vi "Test Script.vi"() -> ()   [LabVIEW 2016, in "PostBuildSupport.lvclass"]
uses:
  PostBuildSupport.lvclass
  PostBuildSupport.lvclass/PostBuildSupport.ctl
panel:
  in  "Output Package File Path":path
  in  "Product Name":string="Multichannel Lockin"
  in  "Package Version":string="2.8.9.18"
  in  "Package Source Folder":path=path "C:/user/patrick/git/Multichannel-Lockin/src"
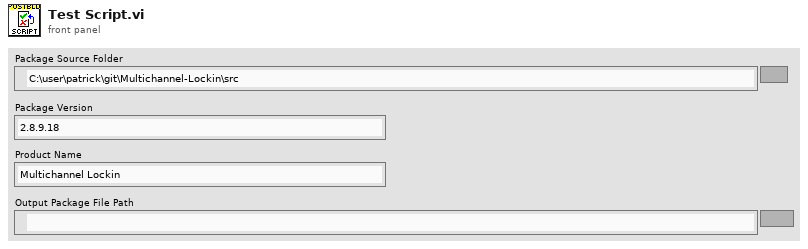
[diagram p1: front panel]
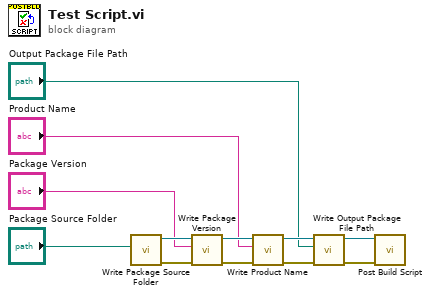
[diagram p0: block diagram]
diagram:
  n1 = call "Write Package Source Folder.vi"("Package Source Folder"="Package Source Folder") -> ("error out"=w11:errorcluster, "PostBuildSupport out"=w12:refnum<class "PostBuildSupport.lvclass">)  [unwired: 9 in]
  n2 = call "Write Package Version.vi"("error in (no error)"=w11, "Package Version"="Package Version", "PostBuildSupport in"=w12) -> ("error out"=w9:errorcluster, "PostBuildSupport out"=w10:refnum<class "PostBuildSupport.lvclass">)  [unwired: 7 in]
  n3 = call "Write Product Name.vi"("error in (no error)"=w9, "Product Name"="Product Name", "PostBuildSupport in"=w10) -> ("error out"=w7:errorcluster, "PostBuildSupport out"=w8:refnum<class "PostBuildSupport.lvclass">)  [unwired: 7 in]
  n4 = call "Write Output Package File Path.vi"("error in (no error)"=w7, "Output Package File Path"="Output Package File Path", "PostBuildSupport in"=w8) -> ("error out"=w5:errorcluster, "PostBuildSupport out"=w6:refnum<class "PostBuildSupport.lvclass">)  [unwired: 7 in]
  n5 = call "Post Build Script.vi"("error in (no error)"=w5, "PostBuildSupport in"=w6) -> ()  [unwired: 9 in, 1 out]
